vi "NXT-HID-Direct.vi"() -> ()   [LabVIEW 2009]
uses:
  <vilib>/NXT/Subs/LVHSConnector.ctl
  <vilib>/NXT/Block Support/NXT_InputPort.ctl
panel:
  in  "Input Port":T1 items=["Port 1", "Port 2", "Port 3", "Port 4"]
  out "NXT dup":T2={"error"={"status"=FALSE, "code"=0, "source"=""}, "address"="", "NXT #"=-1, "Show Error"=TRUE}
  in  "NXT":T2={"error"={"status"=FALSE, "code"=0, "source"=""}, "address"="", "NXT #"=-1, "Show Error"=TRUE}
  in  "Text Data":string="NXTHID is writing this ...."
  in  "Keydata":u8=58 caption="keydata" format="%x"
  in  "Key Modifier":i8(ring) items=["None"=0, "Left Control"=1, "Left Shift"=2, "Left Alt"=4, "Left GUI"=8, "Right Control"=16, "Right Shift"=32, "Right Alt"=64, "Right GUI"=-128]
  in  "Transmit Mode:":u8(ring) caption="Transmit_mode" items=["Direct Keyboard data", "Ascii Text data"]
  # "mindsensors.com\nCopyright (c) 2009 by mindsensors.com\nEmail: info (<at>) mindsensors (<dot>) com\n\nThis program is free software. You can redistribute it and/or modify\nit under the terms of the GNU General Public License as published by\nthe Free Software Foundation; version 3 of the License.\nRead the license at: http://www.gnu.org/licenses/gpl.txt"
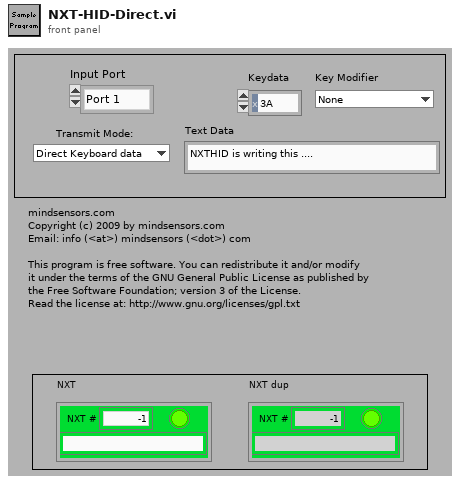
[diagram p1: front panel]
types:
  T1 = typedef "NXT_InputPort.ctl" = u8
  T2 = typedef "LVHSConnector.ctl" = cluster{"error":errorcluster, "address":string, "NXT #":i32, "Show Error":bool}
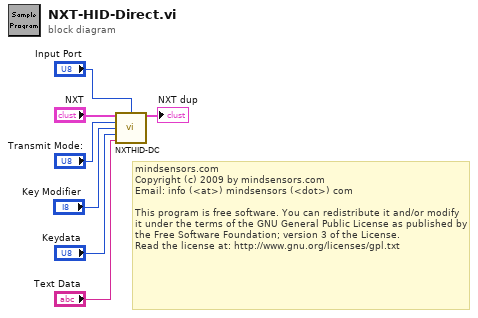
[diagram p0: block diagram]
diagram:
  # "mindsensors.com\nCopyright (c) 2009 by mindsensors.com\nEmail: info (<at>) mindsensors (<dot>) com\n\nThis program is free software. You can redistribute it and/or modify\nit under the terms of the GNU General Public License as published by\nthe Free Software Foundation; version 3 of the License.\nRead the license at: http://www.gnu.org/licenses/gpl.txt"
  n1 = call "NXTHID-DC.vi"("NXT"="NXT", "Input Port"="Input Port", "Transmit Mode"="Transmit Mode:", "Key Modifier"="Key Modifier", "Keydata"="Keydata", "Text Data"="Text Data") -> ("NXT dup"=→"NXT dup":T2)  [unwired: 8 in, 1 out]
